vi "Init DB.vi"(8 "error in (no error)":errorcluster, 11 "SOL-Server in":refnum<class "SOL-Server.lvclass">) -> (0 "error out":errorcluster, 3 "SOL-Server out":refnum<class "SOL-Server.lvclass">)   [LabVIEW 2020, in "Summer of LabVIEW.lvlib" / "SOL-Server.lvclass"]
uses:
  SOL-Server.lvclass
  SOL-Server.lvclass/SOL-Server.ctl
  SQLite/SQLite.lvclass
  Submission DB/Submission DB.lvclass
  Challenge DB/Challenge DB.lvclass
  User DB/User DB.lvclass
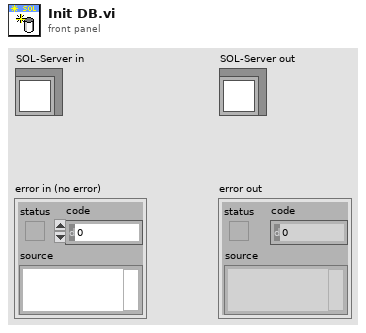
[diagram p1: front panel]
types:
  T1 = typedef "Summer of LabVIEW.lvlib/SOL-Server.lvclass/Paths.ctl" = cluster{"Web Root":path, "Sessions":path, "Config":path, "SQLite DB File":path}
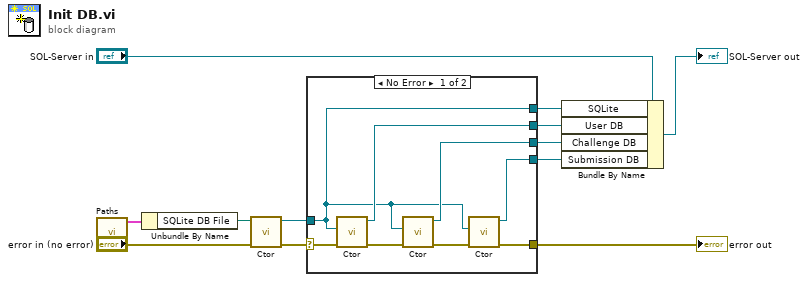
[diagram p0: block diagram]
diagram:
  n1 = call "Paths.vi"() -> ("Paths"=w10:T1)  [unwired: 11 in]
  n2 = Unbundle By Name(w10) -> ("SQLite DB File"=w9:path)
  n3 = call "Ctor.vi"("error in (no error)"="error in (no error)", "DB File"=w9) -> ("error out"=w7:errorcluster, "SQLite out"=w4:refnum<class "SQLite.lvclass">)  [unwired: 8 in]
  n4 = case shown="No Error" w7 {
    selector: w7 -> [w20 w21]
    tunnel: [w19 _] -> w6
    tunnel: [w17 _] -> w5
    tunnel: w4 -> [w13 _]
    tunnel: [w15 _] -> w3
    tunnel: [w14 w21] -> w2
    tunnel: [w13 _] -> w1
    frame No Error {
      n5 = call "Ctor.vi"("error in (no error)"=w20, "SQLite"=w13) -> ("error out"=w18:errorcluster, "User DB out"=w19:refnum<class "User DB.lvclass">)  [unwired: 8 in]
      n6 = call "Ctor.vi"("error in (no error)"=w18, "SQLite"=w13) -> ("error out"=w16:errorcluster, "Challenge DB out"=w17:refnum<class "Challenge DB.lvclass">)  [unwired: 8 in]
      n7 = call "Ctor.vi"("error in (no error)"=w16, "SQLite"=w13) -> ("error out"=w14:errorcluster, "Submission DB out"=w15:refnum<class "Submission DB.lvclass">)  [unwired: 8 in]
    }
    frame Error {
    }
  }
  "error out" <- w2
  n8 = Bundle By Name(cluster="SOL-Server in", "SQLite"=w1, "User DB"=w6, "Challenge DB"=w5, "Submission DB"=w3) -> (→"SOL-Server out":refnum<class "SOL-Server.lvclass">)
